vi "Vision - Dimensions Store.vi"(4 "Page":u8, 6 "Vision Settings":T1 {"Dist/Page" items=["Blue (M)/Black (C)", "Red (M)/Green (C)"]}, 7 "Command":T5, 8 "error in (no error)":errorcluster, 9 "Image Distances _L":dbl[](array[numeric]), 10 "Inc/page (km)":dbl, 11 "Dist/Page Index":T2 caption="Value" items=["Blue (M)/Black (C)", "Red (M)/Green (C)"]) -> (0 "error out":errorcluster, 1 "# of Thumbnails":i32, 2 "Dist/Page (km)":dbl, 3 "Array of ThumbNails":i32[](array[numeric]))   [LabVIEW 2024]
uses:
  Controls/Vision - Dist Per Page.ctl
  Controls/Vision - Image Dimension Command.ctl
  Controls/Vision - Reporting Settings.ctl
  Controls/Vision - Section.ctl
  Buttons/Bin.ctl
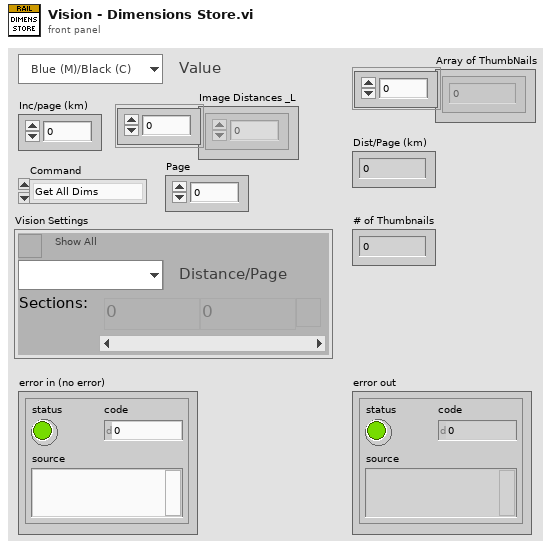
[diagram p1: front panel]
types:
  T1 = typedef "Vision - Reporting Settings.ctl" = cluster{"Show All?":bool, "Dist/Page":T2, "Sections":T3[]}
  T2 = typedef "Vision - Dist Per Page.ctl" = u16
  T3 = typedef "Vision - Section.ctl" = cluster{"From":dbl, "To":dbl, "Discard":T4}
  T4 = typedef "Bin.ctl" = bool
  T5 = typedef "Vision - Image Dimension Command.ctl" = enum16{"Get All Dims", "Get # of Images"}
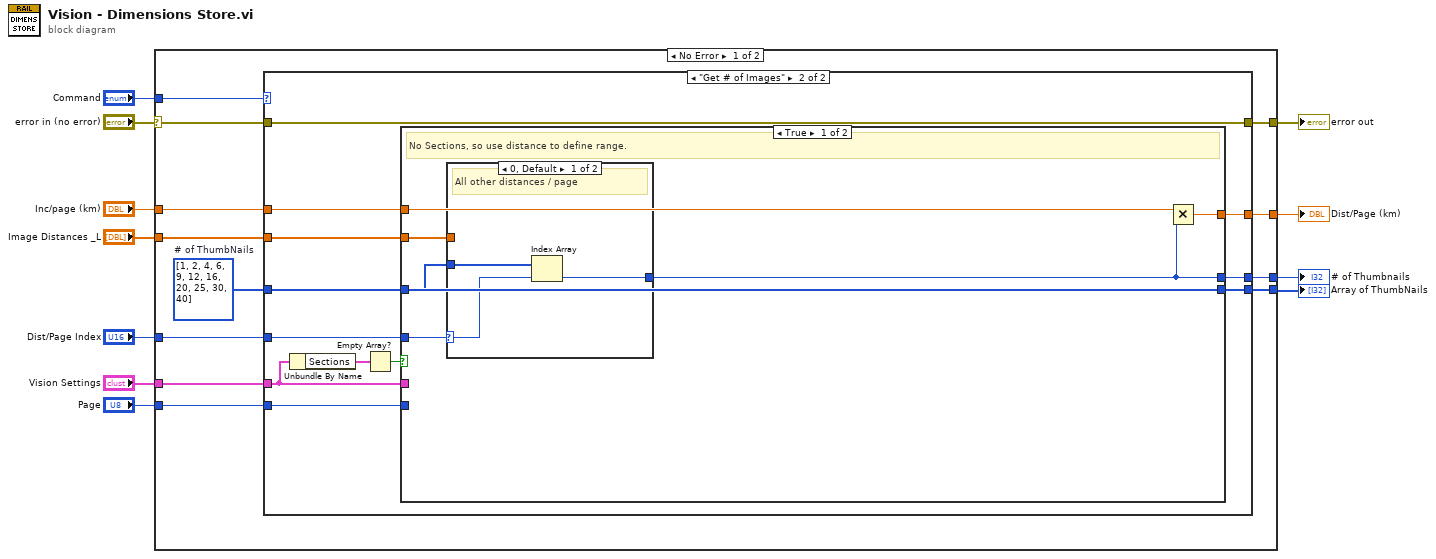
[diagram p0: block diagram]
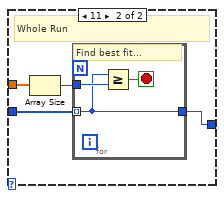
[diagram p3: hidden frame]
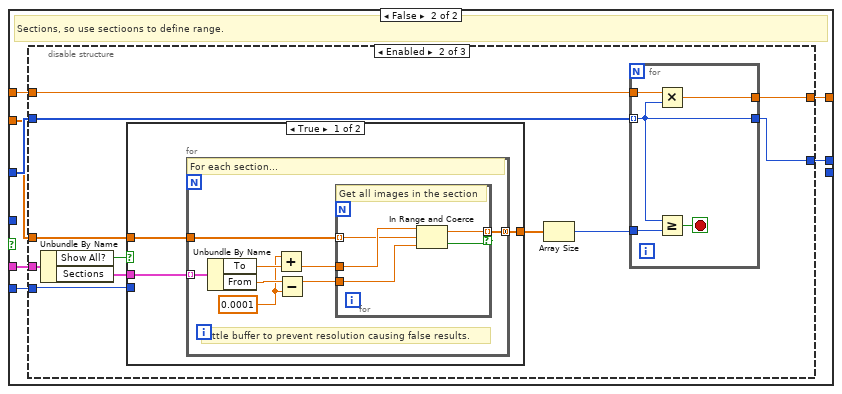
[diagram p4: hidden frame]
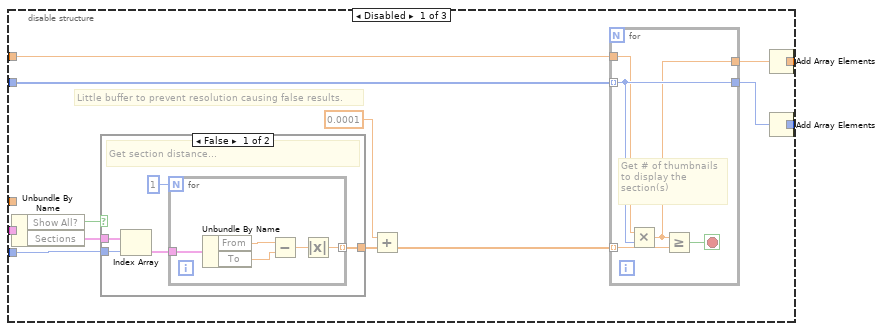
[diagram p5: hidden frame]
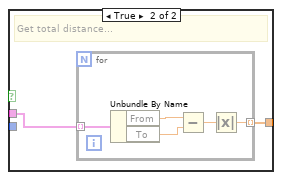
[diagram p6: hidden frame]
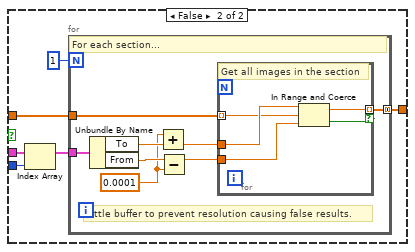
[diagram p7: hidden frame]
diagram:
  n1 = case shown="No Error" "error in (no error)" {
    selector: "error in (no error)" -> [w22 w146]
    tunnel: [w18 _] -> w4
    tunnel: [w23 w146] -> w6
    tunnel: "Command" -> [w21 _]
    tunnel: "Inc/page (km)" -> [w20 _]
    tunnel: "Dist/Page Index" -> [w19 _]
    tunnel: [w16 _] -> w10
    tunnel: [w15 _] -> w11
    tunnel: "Vision Settings" -> [w14 _]
    tunnel: "Page" -> [w13 _]
    tunnel: "Image Distances _L" -> [w12 _]
    frame No Error {
      w17 = i32[] [1, 2, 4, 6, 9, 12, 16, 20, 25, 30, 40]  # # of ThumbNails
      n2 = case shown="\"Get # of Images\"" w21 {
        tunnel: [w25 w36] -> w23
        tunnel: w22 -> [w25 w36]
        tunnel: w20 -> [_ w33]
        tunnel: w19 -> [_ w35]
        tunnel: [w24 w27] -> w18
        tunnel: w17 -> [w24 w27]
        tunnel: [_ w34] -> w16
        tunnel: [_ w32] -> w15
        tunnel: w14 -> [_ w29]
        tunnel: w13 -> [_ w28]
        tunnel: w12 -> [_ w26]
        frame "Get All Dims", Default {
        }
        frame "Get # of Images" {
          n3 = Unbundle By Name(w29) -> ("Sections"=w31:T3[])
          n4 = Empty Array?(array=w31) -> (empty?=w30:bool)
          n5 = case shown="True" w30 {
            tunnel: w27 -> [w42 w56]
            tunnel: w35 -> [w38 _]
            tunnel: [w41 w54] -> w34
            tunnel: w33 -> [w40 w57]
            tunnel: [w39 w55] -> w32
            tunnel: w29 -> [_ w59]
            tunnel: w28 -> [_ w58]
            tunnel: w27 -> [_ _]
            tunnel: w26 -> [w37 w53]
            frame True {
              # "No Sections, so use distance to define range."
              n6 = case shown="0, Default" w38 {
                selector: w38 -> [w43 _]
                tunnel: w42 -> [w45 w47]
                tunnel: [w44 w46] -> w41
                tunnel: w37 -> [_ w49]
                frame 0, Default {
                  # "All other distances / page"
                  n7 = Index Array(array=w45, index=w43) -> (element=w44:i32)
                }
                frame 11 {
                  # "Whole Run"
                  n8 = Array Size(array=w49) -> (size(s)=w48:i32)
                  n9 = for {
                    tunnel: w48 -> [w52]
                    tunnel: w47 -> [w50] mode=indexing
                    tunnel: [w50] -> w46
                    stop <- w51 stop-if-true
                    # "Find best fit..."
                    n10 = Greater Or Equal?(x=w50, y=w52) -> (x >= y?=w51:bool)
                  }
                }
              }
              n11 = Multiply(x=w40, y=w41) -> (x*y=w39:dbl)
            }
            frame False {
              # "Sections, so use sectioons to define range."
              n12 = disable-structure shown="Enabled" {
                disable-tunnel: w59 -> [w72 w105 _]
                disable-tunnel: w58 -> [w69 w95 _]
                disable-tunnel: w57 -> [w68 w104 _]
                disable-tunnel: w56 -> [w67 w103 _]
                disable-tunnel: [w62 w97 _] -> w55
                disable-tunnel: [w60 w96 _] -> w54
                disable-tunnel: w53 -> [_ w100 _]
                frame Disabled {
                  # "Little buffer to prevent resolution causing false results."
                  n13 = Unbundle By Name(w72) -> ("Show All?"=w71:bool, "Sections"=w70:T3[])
                  n14 = case shown="False" w71 {
                    tunnel: w70 -> [w82 w89]
                    tunnel: w69 -> [w81 _]
                    tunnel: [w78 w88] -> w66
                    frame False {
                      # "Get section distance..."
                      n15 = Index Array(array=w82, index=w81) -> (element=w79:T3)
                      n16 = for {
                        N: 1 -> [_]
                        tunnel: w79 -> [w87]
                        tunnel: [w83] -> w78 mode=indexing
                        n17 = Unbundle By Name(w87) -> ("From"=w86:dbl, "To"=w85:dbl)
                        n18 = Subtract(x=w86, y=w85) -> (x-y=w84:dbl)
                        n19 = Absolute Value(x=w84) -> (abs(x)=w83:dbl)
                      }
                    }
                    frame True {
                      # "Get total distance..."
                      n20 = for {
                        tunnel: w89 -> [w94] mode=indexing
                        tunnel: [w90] -> w88 mode=indexing
                        n21 = Unbundle By Name(w94) -> ("From"=w93:dbl, "To"=w92:dbl)
                        n22 = Subtract(x=w93, y=w92) -> (x-y=w91:dbl)
                        n23 = Absolute Value(x=w91) -> (abs(x)=w90:dbl)
                      }
                    }
                  }
                  n24 = Add(x=0.0001 ("y"), y=w66) -> (x+y=w65:dbl[])
                  n25 = for {
                    tunnel: w68 -> [w74]
                    tunnel: w67 -> [w75] mode=indexing
                    tunnel: w65 -> [w77] mode=indexing
                    tunnel: [w75] -> w61
                    tunnel: [w73] -> w63
                    stop <- w76 stop-if-true
                    # "Get # of thumbnails\nto display the\nsection(s)"
                    n26 = Multiply(x=w74, y=w75) -> (x*y=w73:dbl)
                    n27 = Greater Or Equal?(x=w73, y=w77) -> (x >= y?=w76:bool)
                  }
                  n28 = Add Array Elements(numeric array=w63) -> (sum=w62:dbl)
                  n29 = Add Array Elements(numeric array=w61) -> (sum=w60:dbl)
                }
                frame Enabled {
                  n30 = Unbundle By Name(w105) -> ("Show All?"=w101:bool, "Sections"=w102:T3[])
                  n31 = case shown="True" w101 {
                    tunnel: w102 -> [w108 w127]
                    tunnel: w100 -> [w107 w126]
                    tunnel: [w106 w125] -> w99
                    tunnel: w95 -> [_ w123]
                    frame True {
                      n32 = for {
                        tunnel: w107 -> [w116]
                        tunnel: w108 -> [w115] mode=indexing
                        tunnel: [w109] -> w106 mode=concatenating
                        w110 = 0.0001 ("y")
                        # "Little buffer to prevent resolution causing false results."
                        # "For each section..."
                        n33 = Unbundle By Name(w115) -> ("To"=w114:dbl, "From"=w113:dbl)
                        n34 = Add(x=w110, y=w114) -> (x+y=w112:dbl)
                        n35 = Subtract(x=w113, y=w110) -> (x-y=w111:dbl)
                        n36 = for {
                          tunnel: w116 -> [w119] mode=indexing
                          tunnel: w112 -> [w121]
                          tunnel: w111 -> [w120]
                          tunnel: [w118] -> w109 mode=indexing if=w117
                          # "Get all images in the section"
                          n37 = In Range and Coerce(upper limit=w121, x=w119, lower limit=w120) -> (coerced(x)=w118:dbl, In Range?=w117:bool)
                        }
                      }
                    }
                    frame False {
                      n38 = Index Array(array=w127, index=w123) -> (element=w124:T3)
                      n39 = for {
                        N: 1 -> [_]
                        tunnel: w126 -> [w135]
                        tunnel: w124 -> [w134]
                        tunnel: [w128] -> w125 mode=concatenating
                        w129 = 0.0001 ("y")
                        # "Little buffer to prevent resolution causing false results."
                        # "For each section..."
                        n40 = Unbundle By Name(w134) -> ("To"=w133:dbl, "From"=w132:dbl)
                        n41 = Add(x=w129, y=w133) -> (x+y=w131:dbl)
                        n42 = Subtract(x=w132, y=w129) -> (x-y=w130:dbl)
                        n43 = for {
                          tunnel: w135 -> [w138] mode=indexing
                          tunnel: w131 -> [w140]
                          tunnel: w130 -> [w139]
                          tunnel: [w137] -> w128 mode=indexing if=w136
                          # "Get all images in the section"
                          n44 = In Range and Coerce(upper limit=w140, x=w138, lower limit=w139) -> (coerced(x)=w137:dbl, In Range?=w136:bool)
                        }
                      }
                    }
                  }
                  n45 = Array Size(array=w99) -> (size(s)=w98:i32)
                  n46 = for {
                    tunnel: w104 -> [w144]
                    tunnel: w103 -> [w141] mode=indexing
                    tunnel: [w141] -> w96
                    tunnel: [w143] -> w97
                    tunnel: w98 -> [w142]
                    stop <- w145 stop-if-true
                    n47 = Multiply(x=w144, y=w141) -> (x*y=w143:dbl)
                    n48 = Greater Or Equal?(x=w141, y=w142) -> (x >= y?=w145:bool)
                  }
                }
                frame Disabled {
                }
              }
            }
          }
        }
      }
    }
    frame Error {
    }
  }
  "Dist/Page (km)" <- w11
  "# of Thumbnails" <- w10
  "error out" <- w6
  "Array of ThumbNails" <- w4
